vi "clearRoot.vi"(8 "error in (no error)":errorcluster, 11 "xceRootNode in":refnum<class "xceRootNode.lvclass">) -> (0 "error out":errorcluster, 3 "xceRootNode out":refnum<class "xceRootNode.lvclass">)   [LabVIEW 2013, in "xceRootNode.lvclass"]
doc: "Clears the root of all of its subnodes, and deletes tag from the tree control."
uses:
  xceRootNode.lvclass
  xceNode/xceNode.lvclass
  xceRootNode.lvclass/xceRootNode.ctl
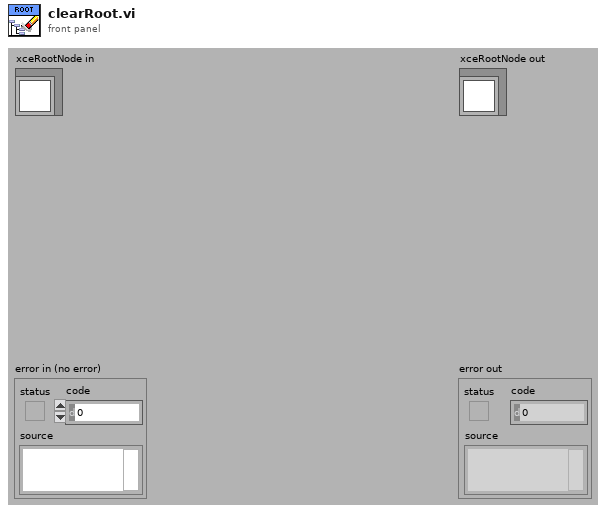
[diagram p1: front panel]
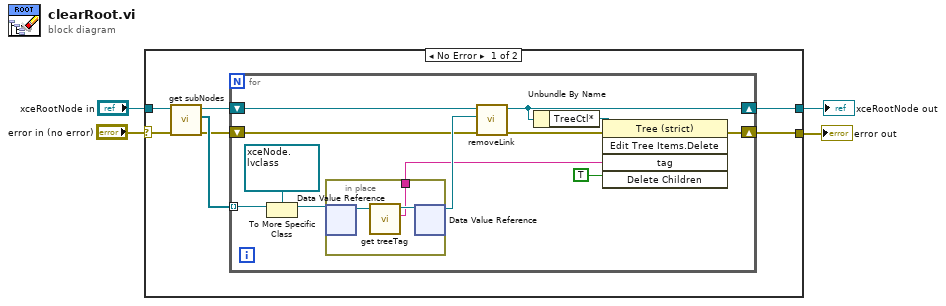
[diagram p0: block diagram]
diagram:
  n1 = case shown="No Error" "error in (no error)" {
    selector: "error in (no error)" -> [w10 w28]
    tunnel: [w5 w28] -> w3
    tunnel: [w6 w27] -> w1
    tunnel: "xceRootNode in" -> [w11 w27]
    frame No Error {
      n2 = call "get subNodes.vi"("error in (no error)"=w10, "xceNode in"=w11) -> ("error out"=w7:errorcluster, "subNodes[]*"=w9:refnum<data-value>[], "xceNode out"=w8:refnum<class "xceRootNode.lvclass">)  [unwired: 7 in]
      n3 = for {
        tunnel: w9 -> [w23] mode=indexing
        shift-right: [w17] -> w6
        shift-left: w8 -> [w20]
        shift-right: [w13] -> w5
        shift-left: w7 -> [w18]
        n4 = To More Specific Class(target class=refnum<data-value> refnum ("data value reference"), reference=w23) -> (specific class reference=w21:refnum<data-value>)  [unwired: 1 in, 1 out]
        n5 = in-place {
          in-place-border: [w24] -> w12
          n6 = in-place-dvr #1(w21) -> (w26:refnum<class "xceNode.lvclass">)  [unwired: 1 out]
          n7 = call "get treeTag.vi"("xceNode in"=w26) -> ("treeTag"=w24:string, "xceNode out"=w25:refnum<class "xceNode.lvclass">)  [unwired: 8 in, 1 out]
          n8 = in-place-dvr #1(w25) -> (w19:refnum<data-value>)  [unwired: 1 out]
        }
        n9 = call "removeLink.vi"("error in (no error)"=w18, "subNode in"=w19, "superNode in"=w20) -> ("error out"=w14:errorcluster, "superNode out"=w17:refnum<class "xceRootNode.lvclass">)  [unwired: 6 in, 1 out]
        n10 = Unbundle By Name(w17) -> ("TreeCtl*"=w16:refnum<vi>)
        n11 = invoke class="Tree (strict)" method="Edit Tree Items.Delete"(reference=w16, error in=w14, "tag"=w12, "Delete Children"=TRUE ("Delete Children?")) -> (error out=w13:errorcluster)  [unwired: 1 in, 4 out]
      }
    }
    frame Error {
    }
  }
  "error out" <- w3
  "xceRootNode out" <- w1
